vi "SaveasTSV.vi"(11 "Graph in":refnum<vi>) -> ()   [LabVIEW 2022 SP3]
uses:
  <vilib>/Utility/error.llb/Trim Whitespace One-Sided.vi
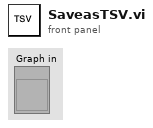
[diagram p1: front panel]
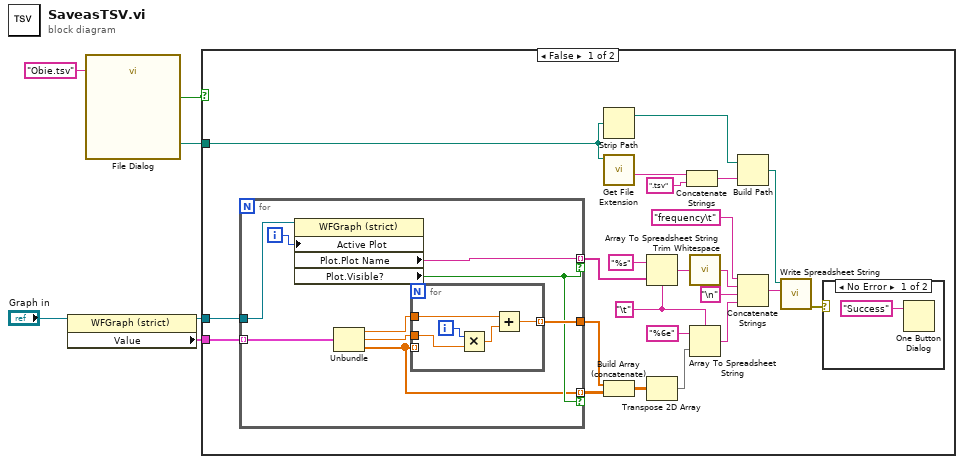
[diagram p0: block diagram]
diagram:
  n1 = property on="Property Node" class="WFGraph (strict)"(reference="Graph in") -> (reference out=w6:refnum<vi>, "Value"=w5:cluster{"x0":dbl, "df":dbl, dbl[]}[])  [unwired: 1 in, 1 out]
  n2 = call "File Dialog"("default name"="Obie.tsv") -> ("selected path"=w3:path, "cancelled"=w2:bool)  [unwired: 11 in, 2 out]
  n3 = case shown="False" w2 {
    tunnel: w6 -> [w19 _]
    tunnel: w5 -> [w10 _]
    tunnel: w3 -> [w7 _]
    frame False {
      w24 = "\t" ("delimiter (Tab)")
      n4 = for {
        tunnel: [w37] -> w12
        tunnel: w10 -> [w36] mode=indexing
        tunnel: [w31] -> w13 mode=indexing if=w32
        tunnel: [w33] -> w14 mode=indexing if=w32
        tunnel: w19 -> [w35]
        i -> [w34]
        n5 = property on="Property Node" class="WFGraph (strict)"(reference=w35, "Active Plot"=w34) -> ("Plot.Plot Name"=w33:string, "Plot.Visible?"=w32:bool)  [unwired: 1 in, 2 out]
        n6 = Unbundle(w36) -> ("x0"=w38:dbl, "df"=w39:dbl, w31:dbl[])
        n7 = for {
          tunnel: w39 -> [w43]
          tunnel: w38 -> [w41]
          tunnel: [w40] -> w37 mode=indexing
          tunnel: w31 -> [_] mode=indexing
          i -> [w42]
          n8 = Multiply(x=w42, y=w43) -> (x*y=w44:dbl)
          n9 = Add(x=w41, y=w44) -> (x+y=w40:dbl)
        }
      }
      n10 = Strip Path(path=w7) -> (stripped path=w28:path)  [unwired: 1 out]
      n11 = call <vilib>:"Get File Extension.vi"("file"=w7) -> ("filename without extension"=w29:string)  [unwired: 6 in, 4 out]
      n12 = Build Array (concatenate)(w12, w13) -> (w17:dbl[][])
      n13 = Array To Spreadsheet String(delimiter (Tab)=w24, array=w14, 3:"%s" ("delimiter (Tab)")) -> (spreadsheet string=w16:string)
      n14 = Transpose 2D Array(2D array=w17) -> (transposed array=w23:dbl[][])
      n15 = Concatenate Strings(w29, ".tsv" ("string")) -> (w25:string)
      n16 = call <vilib>:"Trim Whitespace.vi"("string"=w16) -> ("trimmed string"=w18:string)  [unwired: 1 in]
      n17 = Array To Spreadsheet String(delimiter (Tab)=w24, array=w23, 3:"%6e" ("format string")) -> (spreadsheet string=w8:string)
      n18 = Build Path(base path=w28, name or relative path=w25) -> (appended path=w27:path)
      n19 = Concatenate Strings("frequency\t" ("delimiter (Tab)"), w18, "\n" ("string"), w8) -> (w20:string)
      n20 = call <vilib>:"Write Spreadsheet String.vi"("spreadsheet string"=w20, "file path (dialog if empty)"=w27) -> ("error out"=w22:errorcluster)  [unwired: 8 in, 1 out]
      n21 = case shown="No Error" w22 {
        frame No Error {
          n22 = One Button Dialog(message="Success") -> ()  [unwired: 1 in, 1 out]
        }
        frame Error {
        }
      }
    }
    frame True {
    }
  }
